vi "Get single ROB cluster infoelement ref.vi"(8 "error in (no error)":errorcluster, 10 "Enum":T2(ring), 11 "ROB infocluster ref":T1) -> (0 "error out":errorcluster, 2 "Element reference":refnum<vi>, 3 "ROB infocluster ref":T1)   [LabVIEW 2016]
uses:
  Typedefs/ROB info refnum.ctl
  Typedefs/ROB display info.ctl
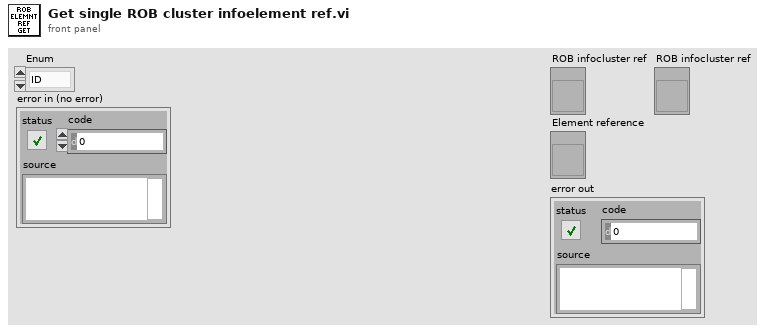
[diagram p1: front panel]
types:
  T1 = typedef "ROB info refnum.ctl" = refnum<vi>
  T2 = enum16{"ID", "Status", "Voltages", "Temp", "Latch count", "VRef", "Trigthres", "MPPC EN?", "Test charge?", "Responding?"}
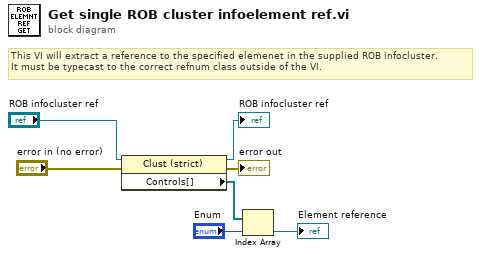
[diagram p0: block diagram]
diagram:
  # "This VI will extract a reference to the specified elemenet in the supplied ROB infocluster.\nIt must be typecast to the correct refnum class outside of the VI."
  n1 = property class="Clust (strict)"(reference="ROB infocluster ref", error in="error in (no error)") -> (reference out=→"ROB infocluster ref":T1, error out=→"error out":errorcluster, "Controls[]"=w7:refnum<vi>[])
  n2 = Index Array(array=w7, index="Enum") -> (element=→"Element reference":refnum<vi>)
